vi "Pr650Initiate 01.vi"(9 "Port":i32(ring) items=["COM1", "COM2"]) -> (1 "string read":string)   [LabVIEW 2009]
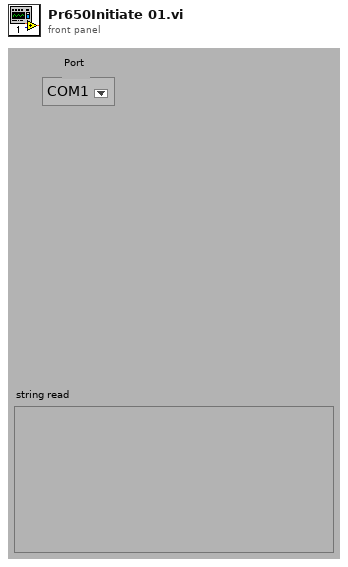
[diagram p1: front panel]
types:
  T1 = cluster{"input XON/XOFF":bool, "input HW Handshake":bool, "input alt HW HShk":bool, "output XON/XOFF":bool, "output HW Handshake":bool, "output alt HW HShk":bool, "XOFF byte":u8, "XON byte":u8, "parity error byte":u16}
  T2 = enum16{"no parity", "odd parity", "even parity", "mark parity", "space parity"}
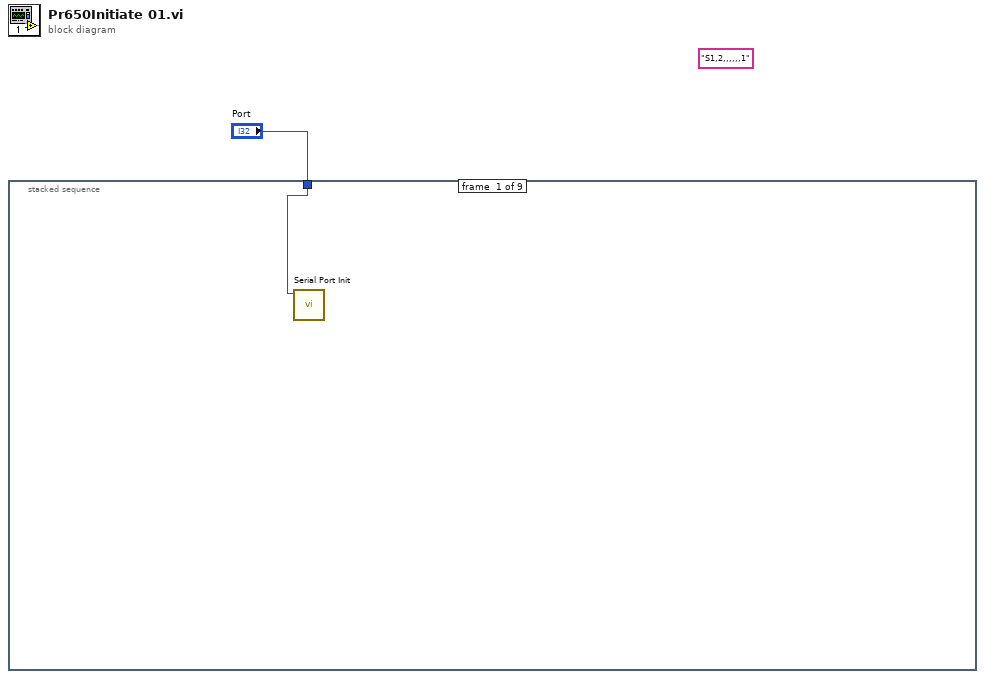
[diagram p0: block diagram]
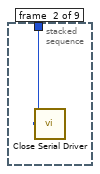
[diagram p2: hidden frame]
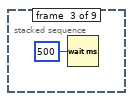
[diagram p3: hidden frame]
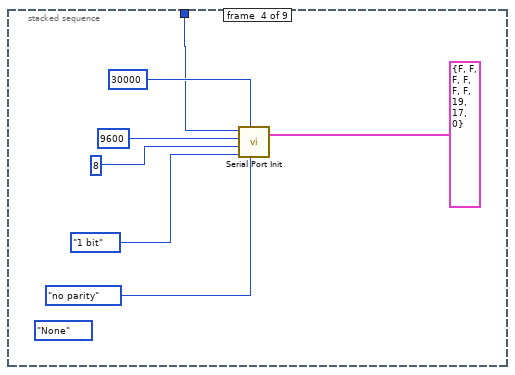
[diagram p4: hidden frame]
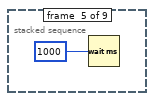
[diagram p5: hidden frame]
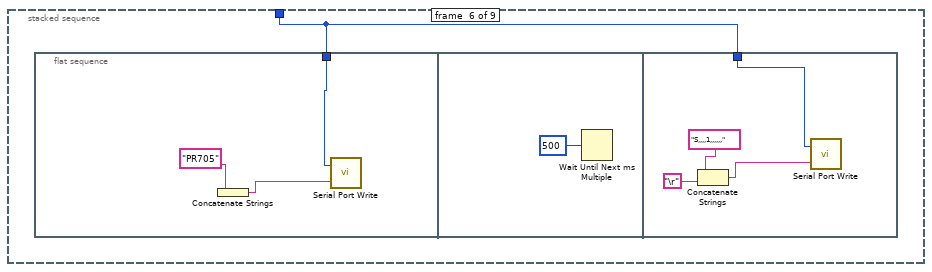
[diagram p6: hidden frame]
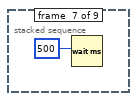
[diagram p7: hidden frame]
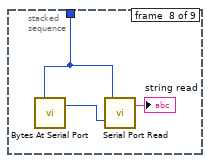
[diagram p8: hidden frame]
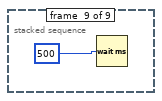
[diagram p9: hidden frame]
diagram:
  (unwired) "S1,2,,,,,,1"
  n1 = stacked-sequence {
    tunnel: "Port" -> [w2 w3 _ w9 _ w13 _ w25 _]
    frame #0 {
      n2 = call <vilib>:"Serial Port Init.vi"("port number"=w2) -> ()  [unwired: 6 in, 1 out]
    }
    frame #1 {
      n3 = call <vilib>:"Close Serial Driver.vi"("port number"=w3) -> ()  [unwired: 1 out]
    }
    frame #2 {
      n4 = Wait (ms)(milliseconds to wait=u32 500) -> ()  [unwired: 1 out]
    }
    frame #3 {
      (unwired) enum16{"None", "Odd", "Even", "Mark", "Space"}."None" ("parity (0:none)")
      n5 = call <vilib>:"Serial Port Init.vi"("flow control etc."=T1 {"input XON/XOFF"=FALSE, "input HW Handshake"=FALSE, "input alt HW HShk"=FALSE, "output XON/XOFF"=FALSE, "output HW Handshake"=FALSE, "output alt HW HShk"=FALSE, "XOFF byte"=19, "XON byte"=17, "parity error byte"=0}, "parity"=T2."no parity" ("parity 2"), "buffer size"=u16 30000 ("buffer size 2"), "stop bits"=enum16{"1 bit", "1.5 bits", "2 bits"}."1 bit" ("stop bits 2"), "data bits"=u16 8 ("data bits 2"), "baud rate"=u32 9600 ("baud rate 2"), "port number"=w9) -> ()  [unwired: 1 out]
    }
    frame #4 {
      n6 = Wait (ms)(milliseconds to wait=1000) -> ()  [unwired: 1 out]
    }
    frame #5 {
      n7 = flat-sequence {
        tunnel: w13 -> [w14]
        tunnel: w13 -> [w18]
        frame #0 {
          n8 = Concatenate Strings("PR705") -> (w15:string)
          n9 = call <vilib>:"Serial Port Write.vi"("string to write"=w15, "port number"=w14) -> ()  [unwired: 1 out]
        }
        frame #1 {
          n10 = Wait Until Next ms Multiple(millisecond multiple=u32 500) -> ()  [unwired: 1 out]
        }
        frame #2 {
          n11 = Concatenate Strings("S,,,,1,,,,,,", "\r") -> (w19:string)
          n12 = call <vilib>:"Serial Port Write.vi"("string to write"=w19, "port number"=w18) -> ()  [unwired: 1 out]
        }
      }
    }
    frame #6 {
      n13 = Wait (ms)(milliseconds to wait=500) -> ()  [unwired: 1 out]
    }
    frame #7 {
      n14 = call <vilib>:"Bytes At Serial Port.vi"("port number"=w25) -> ("byte count"=w24:u32)  [unwired: 1 out]
      n15 = call <vilib>:"Serial Port Read.vi"("requested byte count"=w24, "port number"=w25) -> ("string read"=→"string read":string)  [unwired: 1 out]
    }
    frame #8 {
      n16 = Wait (ms)(milliseconds to wait=500) -> ()  [unwired: 1 out]
    }
  }
